vi "SubVI_CoEIndexRead.vi"(8 "error in (no error)":errorcluster, 9 "SubIndex":u8, 10 "Index":u16, 11 "Device address":string) -> (0 "error out":errorcluster, 3 "output cluster":T3 {"Object Entry"."Index" format="%x"; "Object Entry"."SubIndex" format="%x"; "Object Entry"."DataType" items=["UNDEFINED"=0, "BOOLEAN"=1, "INTEGER8"=2, "INTEGER16"=3, "INTEGER32"=4, "UNSIGNED8"=5, "UNSIGNED16"=6, "UNSIGNED32"=7, "REAL32"=8, "VISIBLE_STRING"=9, "OCTET_STRING"=10, "UNICODE_STRING"=11, "TIME_OF_DAY"=12, "TIME_DIFFERENCE"=13, "DOMAIN"=15, "INTEGER24"=16, "REAL64"=17, "INTEGER40"=18, "INTEGER48"=19, "INTEGER56"=20, "INTEGER64"=21, "UNSIGNED40"=23, "UNSIGNED48"=24, "UNSIGNED56"=25, "UNSIGNED64"=26, "GUID"=29, "BYTE"=30, "BITARR8"=45, "BITARR16"=46, "BITARR32"=47, "PDO_MAPPING"=33, "IDENTITY"=35, "COMMAND_PAR"=37, "SYNC_PAR"=41, "BIT1"=48, "BIT2"=49, "BIT3"=50, "BIT4"=51, "BIT5"=52, "BIT6"=53, "BIT7"=54, "BIT8"=55, "ENUM"=2048]})   [LabVIEW 2022 SP3, in "EtherCAT_Library.lvlib"]
doc: "This SubVI takes in a EtherCAT Device Address as input, in the format AMSNetID:EtherCATAddress, for example 127.0.0.0.1.1:1001\n\nThe Index and SubIndex inputs allow you to specify the CoE Index of the target to be read\n\nThe output is a cluster containing the Name, details and data from the CoE index."
uses:
  EtherCAT_Library.lvlib
  <userlib>/Beckhoff-LabVIEW-Interface/_DependsOn/TypeDefs/Utilities/CoE Object Entry.ctl
  <userlib>/Beckhoff-LabVIEW-Interface/_DependsOn/TypeDefs/Utilities/CoE Object DataType.ctl
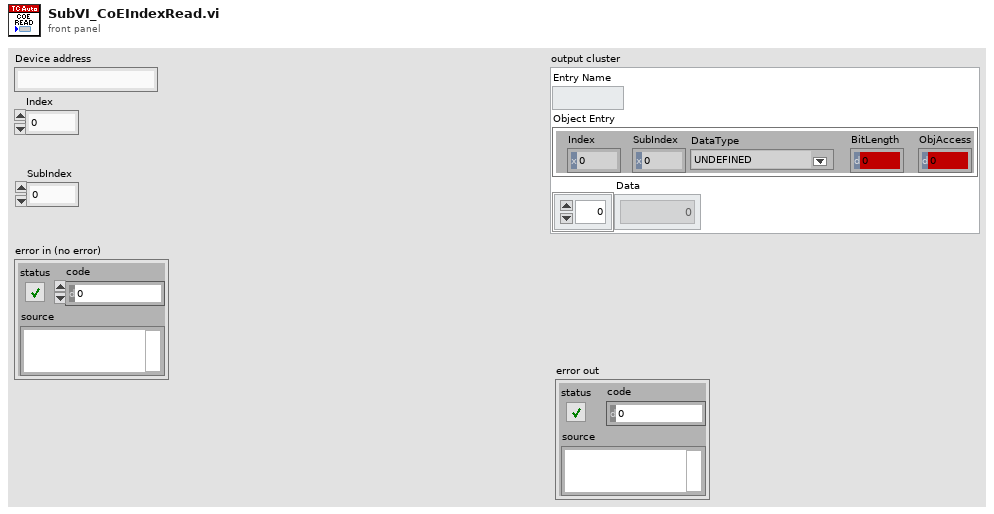
[diagram p1: front panel]
types:
  T1 = typedef "CoE Object Entry.ctl" = cluster{"Index":u16, "SubIndex":u8, "ValueInfo":u8, "DataType":T2, "BitLength":u16, "ObjAccess":u16}
  T2 = typedef "CoE Object DataType.ctl" = u16
  T3 = cluster{"Entry Name":string, "Object Entry":T1, "Data":u8[]}
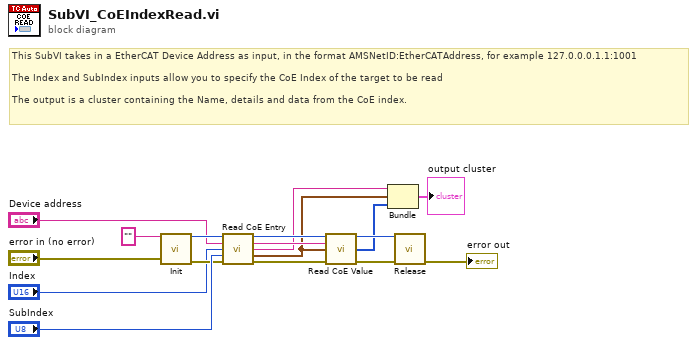
[diagram p0: block diagram]
diagram:
  # "This SubVI takes in a EtherCAT Device Address as input, in the format AMSNetID:EtherCATAddress, for example 127.0.0.0.1.1:1001\n\nThe Index and SubIndex inputs allow you to specify the CoE Index of the target to be read\n\nThe output is a cluster containing the Name, details and data from the CoE index."
  n1 = call <userlib>:"Init.vi"("XMLDescription"="", "error in (no error)"="error in (no error)") -> ("Handle"=w10:u32, "error out"=w9:errorcluster)  [unwired: 9 in, 3 out]
  n2 = call <userlib>:"Read CoE Entry.vi"("Handle"=w10, "Device Address"="Device address", "Index"="Index", "SubIndex"="SubIndex", "error constant"=w9) -> ("Handle"=w15:u32, "Device Address"=w14:string, "Entry Name"=w6:string, "Object Entry"=w5:T1, "error out"=w13:errorcluster)  [unwired: 6 in]
  n3 = call <userlib>:"Read CoE Value.vi"("Handle"=w15, "Device Address"=w14, "CoE Entry"=w5, "error constant"=w13) -> ("Handle"=w11:u32, "Data"=w4:u8[], "error out"=w12:errorcluster)  [unwired: 8 in, 1 out]
  n4 = Bundle("Entry Name"=w6, "Object Entry"=w5, "Data"=w4) -> (→"output cluster":T3)  [unwired: 1 in]
  n5 = call <userlib>:"Release.vi"("Handle"=w11, "error in (no error)"=w12) -> ("error out"=→"error out":errorcluster)  [unwired: 13 in]
